vi "Layout Ports.vi"(8 "error in (no error)":errorcluster, 11 "Node in":refnum<class "FSM.Node.lvclass">) -> (0 "error out":errorcluster, 3 "Node out":refnum<class "FSM.Node.lvclass">)   [LabVIEW 2015, in "FSM.Node.lvclass"]
uses:
  FSM.Node.lvclass
  FSM.Node.lvclass/FSM.Node.ctl
  FSM.Port/FSM.Port.lvclass
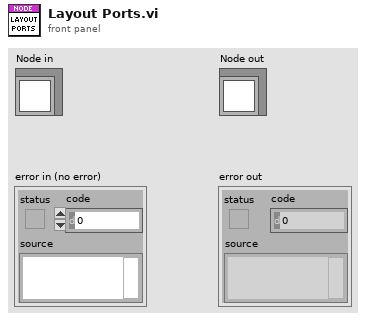
[diagram p1: front panel]
types:
  T1 = typedef "FSM.Node.lvclass/Shape.ctl" = enum16{"Default", "Start", "Action", "End"}
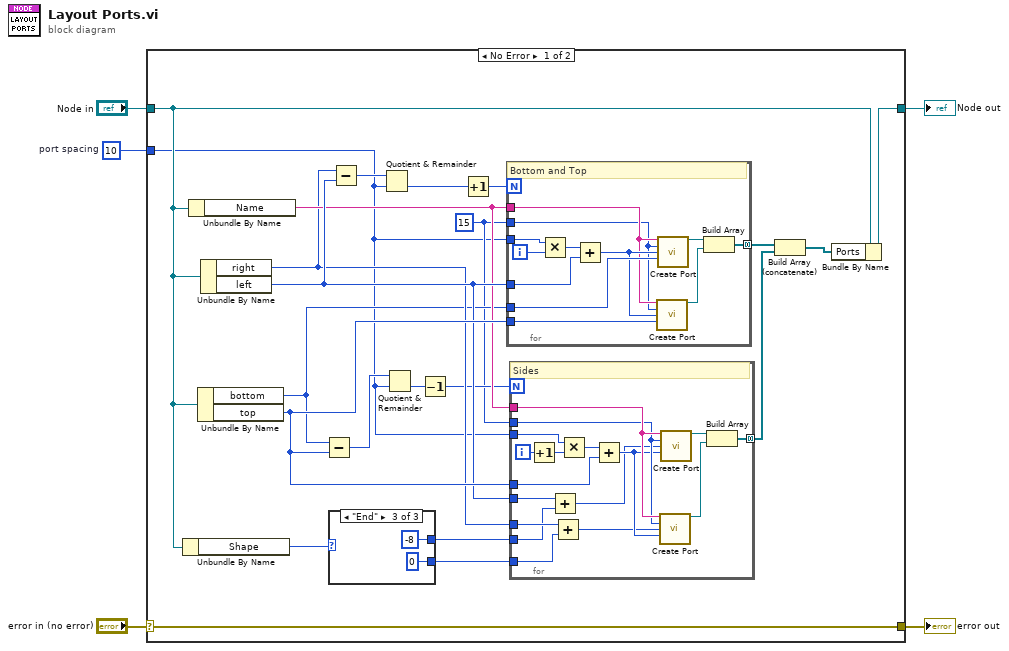
[diagram p0: block diagram]
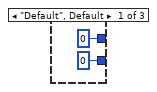
[diagram p2: hidden frame]
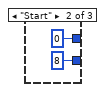
[diagram p3: hidden frame]
diagram:
  w1 = 10  # port spacing
  n1 = case shown="No Error" "error in (no error)" {
    selector: "error in (no error)" -> [w27 w64]
    tunnel: [w27 w64] -> w4
    tunnel: [w23 w63] -> w2
    tunnel: "Node in" -> [w11 w63]
    tunnel: w1 -> [w6 _]
    frame No Error {
      w7 = 15
      n2 = Unbundle By Name(w11) -> ("Shape"=w10:T1)
      n3 = Unbundle By Name(w11) -> ("Name"=w19:string)
      n4 = Unbundle By Name(w11) -> ("bottom"=w17:i16, "top"=w21:i16)
      n5 = Unbundle By Name(w11) -> ("right"=w18:i16, "left"=w20:i16)
      n6 = Subtract(x=w17, y=w21) -> (x-y=w25:i16)
      n7 = case shown="\"End\"" w10 {
        tunnel: [0 8 0] -> w9
        tunnel: [0 0 -8] -> w8
        frame "Default", Default {
        }
        frame "Start" {
        }
        frame "End" {
        }
      }
      n8 = Subtract(x=w18, y=w20) -> (x-y=w26:i16)
      n9 = Quotient & Remainder(x=w26, y=w6) -> (floor(x/y)=w24:i32)  [unwired: 1 out]
      n10 = Quotient & Remainder(x=w25, y=w6) -> (floor(x/y)=w22:i32)  [unwired: 1 out]
      n11 = Decrement(x=w22) -> (x-1=w12:i32)
      n12 = Increment(x=w24) -> (x+1=w13:i32)
      n13 = for {
        N: w13 -> [_]
        tunnel: w7 -> [w52]
        tunnel: w21 -> [w57]
        tunnel: w20 -> [w60]
        tunnel: w17 -> [w59]
        tunnel: [w54] -> w16 mode=concatenating
        tunnel: w19 -> [w53]
        tunnel: w6 -> [w51]
        i -> [w62]
        # "Bottom and Top"
        n14 = Multiply(x=w51, y=w62) -> (x*y=w61:i32)
        n15 = Add(x=w61, y=w60) -> (x+y=w58:i32)
        n16 = call "Create Port.vi"("Node name"=w53, "size"=w52, "x"=w58, "y"=w57) -> ("FSM.Port"=w55:refnum<class "FSM.Port.lvclass">)  [unwired: 11 in]
        n17 = call "Create Port.vi"("Node name"=w53, "size"=w52, "x"=w58, "y"=w59) -> ("FSM.Port"=w56:refnum<class "FSM.Port.lvclass">)  [unwired: 11 in]
        n18 = Build Array(w56, w55) -> (w54:refnum<class "FSM.Port.lvclass">[])
      }
      n19 = for {
        N: w12 -> [_]
        tunnel: w7 -> [w43]
        tunnel: w21 -> [w48]
        tunnel: [w45] -> w15 mode=concatenating
        tunnel: w19 -> [w44]
        tunnel: w20 -> [w42]
        tunnel: w18 -> [w41]
        tunnel: w9 -> [w36]
        tunnel: w8 -> [w35]
        tunnel: w6 -> [w34]
        i -> [w50]
        # "Sides"
        n20 = Increment(x=w50) -> (x+1=w39:i32)
        n21 = Add(x=w42, y=w35) -> (x+y=w38:i32)
        n22 = Add(x=w41, y=w36) -> (x+y=w37:i32)
        n23 = Multiply(x=w34, y=w39) -> (x*y=w49:i32)
        n24 = Add(x=w49, y=w48) -> (x+y=w40:i32)
        n25 = call "Create Port.vi"("Node name"=w44, "size"=w43, "x"=w37, "y"=w40) -> ("FSM.Port"=w46:refnum<class "FSM.Port.lvclass">)  [unwired: 11 in]
        n26 = call "Create Port.vi"("Node name"=w44, "size"=w43, "x"=w38, "y"=w40) -> ("FSM.Port"=w47:refnum<class "FSM.Port.lvclass">)  [unwired: 11 in]
        n27 = Build Array(w47, w46) -> (w45:refnum<class "FSM.Port.lvclass">[])
      }
      n28 = Build Array (concatenate)(w16, w15) -> (w14:refnum<class "FSM.Port.lvclass">[])
      n29 = Bundle By Name(cluster=w11, "Ports"=w14) -> (w23:refnum<class "FSM.Node.lvclass">)
    }
    frame Error {
    }
  }
  "error out" <- w4
  "Node out" <- w2
